vi "Volts to FXP Codes.vi"(0 "scaling coefficients":T1[](array[typedef]), 5 "channel index":u8, 7 "level (V)":dbl) -> (4 "codes":fxp<+/-,18,1> format="%.18g")   [LabVIEW 2021, in "Device Session.lvclass"]
uses:
  Device Session.lvclass
  <instrlib>/_niInstr/Multirecord Acquisition/Interface/v1/Host/Public/Scaling Coefficient.ctl
  <instrlib>/_niInstr/Multirecord Acquisition/Interface/v1/Host/niInstr Multirecord Acquisition v1 Host.lvclass
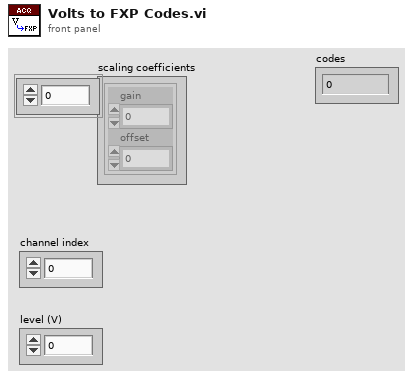
[diagram p1: front panel]
types:
  T1 = typedef "niInstr Multirecord Acquisition v1 Host.lvclass/Scaling Coefficient.ctl" = cluster{"gain":dbl, "offset":dbl}
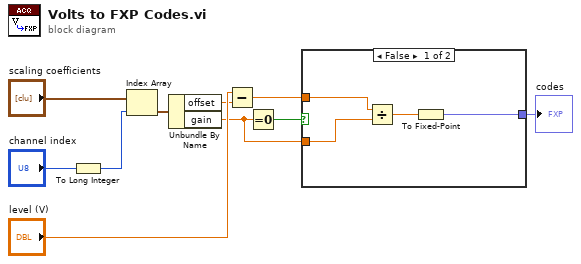
[diagram p0: block diagram]
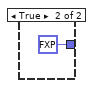
[diagram p2: hidden frame]
diagram:
  n1 = To Long Integer(number="channel index") -> (32bit integer=w1:i32)
  n2 = Index Array(array="scaling coefficients", index=w1) -> (element=w8:T1)
  n3 = Unbundle By Name(w8) -> ("offset"=w7:dbl, "gain"=w4:dbl)
  n4 = Subtract(x="level (V)", y=w7) -> (x-y=w9:dbl)
  n5 = Equal To 0?(x=w4) -> (x = 0?=w6:bool)
  n6 = case shown="False" w6 {
    tunnel: w9 -> [w14 _]
    tunnel: [w12 fxp<+/-,18,1> 0.0] -> w5
    tunnel: w4 -> [w11 _]
    frame False {
      n7 = Divide(x=w14, y=w11) -> (x/y=w13:dbl)
      n8 = To Fixed-Point(number=w13) -> (fixed-point=w12:fxp<+/-,18,1>)  [unwired: 1 in]
    }
    frame True {
    }
  }
  "codes" <- w5
